vi "MicroSlide-Parser.vi"(7 "String":string) -> (6 "Answer":string, 10 "Leftovers":string, 13 "Received":bool)   [LabVIEW 2019]
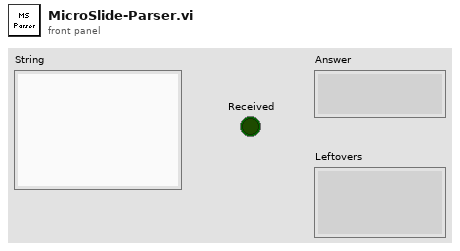
[diagram p1: front panel]
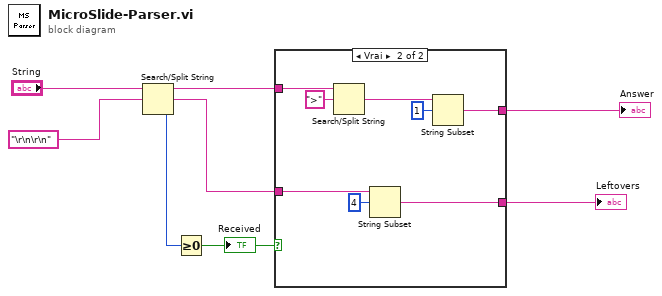
[diagram p0: block diagram]
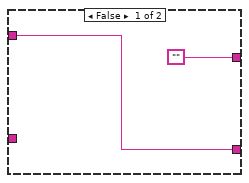
[diagram p2: hidden frame]
diagram:
  n1 = Search/Split String(string="String", search string/char (-)="\r\n\r\n") -> (substring before match=w5:string, match + rest of string=w4:string, offset of match=w7:i32)  [unwired: 1 in]
  n2 = Greater Or Equal To 0?(x=w7) -> (x >= 0?=w3:bool)
  "Received" <- w3
  n3 = case shown="Vrai" w3 {
    tunnel: w5 -> [w9 w18]
    tunnel: w4 -> [_ w13]
    tunnel: ["" ("String") w15] -> w2
    tunnel: [w9 w12] -> w1
    frame False {
    }
    frame True {
      n4 = Search/Split String(string=w18, search string/char (-)=">") -> (match + rest of string=w11:string)  [unwired: 1 in, 2 out]
      n5 = String Subset(string=w13, offset (0)=4) -> (substring=w12:string)  [unwired: 1 in]
      n6 = String Subset(string=w11, offset (0)=1) -> (substring=w15:string)  [unwired: 1 in]
    }
  }
  "Answer" <- w2
  "Leftovers" <- w1
